vi "IIR Filter PtByPt.vi"(2 "initialize":bool, 3 "Forward Coefficients":dbl[](array[numeric]), 4 "Reverse Coefficients":dbl[](array[numeric]), 5 "x":dbl format="%0.2f") -> (0 "error":i32, 1 "Filtered x":dbl format="%0.2f")   [LabVIEW 2020, in "NI_PtbyPt.lvlib"]
doc: "Filters <B>x</B> using the direct form IIR filter specified by <B>Reverse Coefficients</B> and <B>Forward Coefficients</B>."
uses:
  NI_PtbyPt.lvlib
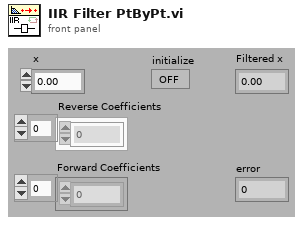
[diagram p1: front panel]
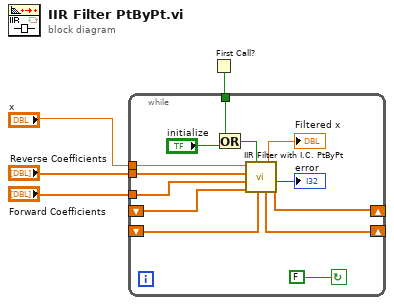
[diagram p0: block diagram]
diagram:
  n1 = First Call?() -> (First Call?: T/F=w1:bool)
  n2 = while {
    tunnel: w1 -> [w6]
    tunnel: "x" -> [w15]
    shift-left: _ -> [w12]
    shift-right: [w11] -> _
    shift-left: _ -> [w14]
    shift-right: [w13] -> _
    tunnel: "Forward Coefficients" -> [w16]
    tunnel: "Reverse Coefficients" -> [w17]
    stop <- FALSE continue-if-true
    n3 = Or(x=w6, y="initialize") -> (x .or. y?=w7:bool)
    n4 = call "IIR Filter with I.C. PtByPt.vi"("Initial Y Conditions"=w12, "initialize"=w7, "Initial X Conditions"=w14, "Forward Coefficients"=w16, "Reverse Coefficients"=w17, "x"=w15) -> ("Final X Conditions"=w13:dbl[], "error"=→"error":i32, "Filtered x"=→"Filtered x":dbl, "Final Y Conditions"=w11:dbl[])  [unwired: 2 in]
  }
